vi "Saved Position Configuration.vi"(10 "Saved Position":dbl[](array[numeric]), 11 "Action":enum16{"Read", "Write"}(ring)) -> (2 "Saved Position":dbl[](array[numeric]))   [LabVIEW 2018, in "Stage Actor.lvlib"]
uses:
  Stage Actor.lvlib
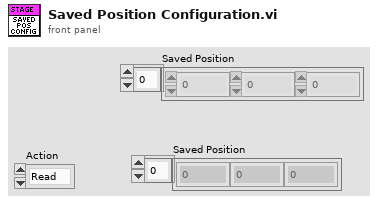
[diagram p1: front panel]
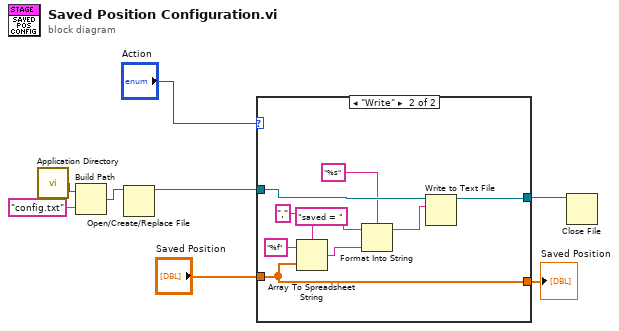
[diagram p0: block diagram]
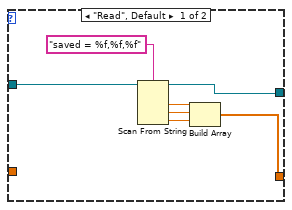
[diagram p2: hidden frame]
diagram:
  n1 = call <vilib>:"Application Directory.vi"() -> ("Application Directory"=w8:path)
  n2 = Build Path(base path=w8, name or relative path="config.txt") -> (appended path=w7:path)
  n3 = Open/Create/Replace File(file path (use dialog)=w7) -> (refnum out=w4:refnum<file>)  [unwired: 5 in, 2 out]
  n4 = case shown="\"Write\"" "Action" {
    tunnel: w4 -> [w15 w24]
    tunnel: [w14 w23] -> w3
    tunnel: [w9 w18] -> w2
    tunnel: "Saved Position" -> [_ w18]
    frame "Read", Default {
      n5 = Scan From String("saved = %f,%f,%f" ("format string"), w15) -> (w14:refnum<file>, output 1=w12:dbl, output 2=w10:dbl, output 3=w11:dbl)  [unwired: 4 in, 1 out]
      n6 = Build Array(w12, w10, w11) -> (w9:dbl[])
    }
    frame "Write" {
      n7 = Array To Spreadsheet String(delimiter (Tab)=",", array=w18, 3:"%f" ("format string")) -> (spreadsheet string=w22:string)
      n8 = Format Into String(format string="%s", initial string="saved = ", w22) -> (resulting string=w19:string)  [unwired: 1 in, 1 out]
      n9 = Write to Text File(file (use dialog)=w24, text=w19) -> (refnum out=w23:refnum<file>)  [unwired: 2 in, 2 out]
    }
  }
  "Saved Position" <- w2
  n10 = Close File(refnum=w3) -> ()  [unwired: 1 in, 2 out]
